vi "EvaluateNode.vi"(8 "error in (no error)":errorcluster, 10 "ToEvaluate in":refnum<data-value>, 11 "Graph in":refnum<class "Graph.lvclass">) -> (0 "error out":errorcluster, 2 "ToEvaluate out":refnum<data-value>, 3 "Graph out":refnum<class "Graph.lvclass">)   [LabVIEW 2014, in "Graph.lvlib" / "Graph.lvclass"]
doc: "Calls the Evaluation method of a node, then applies the value to the node, then sets the ToSortBy so it can be placed in OPEN."
uses:
  <userlib>/AdvancedDataStructures/ClassBased/Graph/Graph.lvclass
  <userlib>/AdvancedDataStructures/ClassBased/GraphNode/GraphNode.lvclass
  <userlib>/AdvancedDataStructures/ClassBased/Common/BasicSortedList/BasicSortedNode/BasicSortedNode.lvclass
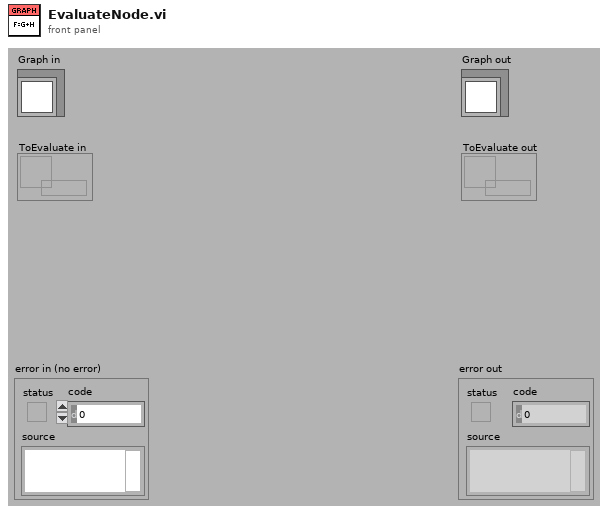
[diagram p1: front panel]
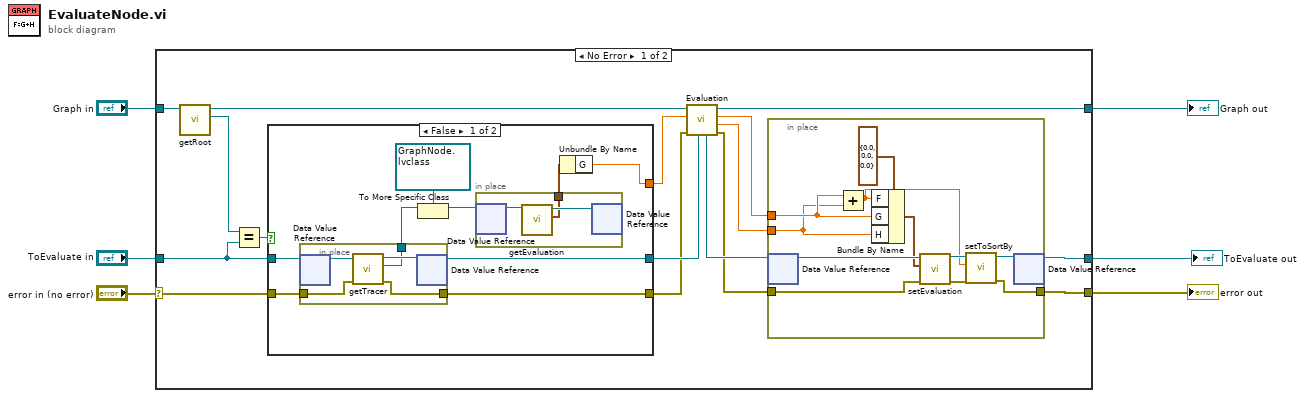
[diagram p0: block diagram]
diagram:
  n1 = case shown="No Error" "error in (no error)" {
    selector: "error in (no error)" -> [w18 w55]
    tunnel: [w8 w55] -> w5
    tunnel: [w7 w54] -> w3
    tunnel: "Graph in" -> [w22 w54]
    tunnel: "ToEvaluate in" -> [w19 w53]
    tunnel: [w9 w53] -> w1
    frame No Error {
      n2 = call <userlib>:"getRoot.vi"("Graph in"=w22) -> ("Root"=w21:refnum<data-value>, "Graph out"=w17:refnum<class "Graph.lvclass">)  [unwired: 8 in, 1 out]
      n3 = Equal?(x=w21, y=w19) -> (x = y?=w20:bool)
      n4 = case shown="False" w20 {
        tunnel: w19 -> [w42 w52]
        tunnel: [w39 w52] -> w15
        tunnel: w18 -> [w41 w51]
        tunnel: [w40 w51] -> w14
        tunnel: [w35 _] -> w16
        frame False {
          n5 = in-place {
            in-place-border: [w48] -> w38
            in-place-border: w41 -> [w47]
            in-place-border: [w46] -> w40
            n6 = in-place-dvr #1(w42) -> (w50:refnum<class "GraphNode.lvclass">)  [unwired: 1 out]
            n7 = call <userlib>:"getTracer.vi"("error in (no error)"=w47, "GraphNode in"=w50) -> ("error out"=w46:errorcluster, "tracer"=w48:refnum<data-value>, "GraphNode out"=w49:refnum<class "GraphNode.lvclass">)  [unwired: 7 in]
            n8 = in-place-dvr #1(w49) -> (w39:refnum<data-value>)  [unwired: 1 out]
          }
          n9 = To More Specific Class(target class=refnum<data-value> refnum ("ToEvaluate in"), reference=w38) -> (specific class reference=w36:refnum<data-value>)  [unwired: 1 in, 1 out]
          n10 = in-place {
            in-place-border: [w43] -> w34
            n11 = in-place-dvr #2(w36) -> (w45:refnum<class "GraphNode.lvclass">)  [unwired: 1 out]
            n12 = call <userlib>:"getEvaluation.vi"("GraphNode in"=w45) -> ("Evaluation"=w43:cluster{"F":dbl, "G":dbl, "H":dbl}, "GraphNode out"=w44:refnum<class "GraphNode.lvclass">)  [unwired: 8 in, 1 out]
            n13 = in-place-dvr #2(w44) -> ()  [unwired: 2 out]
          }
          n14 = Unbundle By Name(w34) -> ("G"=w35:dbl)
        }
        frame True {
        }
      }
      n15 = call-dynamic "Evaluation.vi"("ToEvaluate in"=w15, "error in (no error)"=w14, "Parents G"=w16, "Graph in"=w17) -> ("error out"=w10:errorcluster, "H"=w11:dbl, "G"=w12:dbl, "Graph out"=w7:refnum<class "Graph.lvclass">, "ToEvaluate out"=w13:refnum<data-value>)  [unwired: 3 in]
      n16 = in-place {
        in-place-border: w12 -> [w32]
        in-place-border: w11 -> [w31]
        in-place-border: w10 -> [w25]
        in-place-border: [w23] -> w8
        n17 = in-place-dvr #3(w13) -> (w30:refnum<class "GraphNode.lvclass">)  [unwired: 1 out]
        n18 = Add(x=w32, y=w31) -> (x+y=w26:dbl)
        n19 = Bundle By Name(cluster=cluster{"F":dbl, "G":dbl, "H":dbl} {"F"=0.0, "G"=0.0, "H"=0.0} ("evaluation"), "F"=w26, "G"=w32, "H"=w31) -> (w29:cluster{"F":dbl, "G":dbl, "H":dbl})
        n20 = call <userlib>:"setEvaluation.vi"("error in (no error)"=w25, "Evaluation"=w29, "GraphNode in"=w30) -> ("error out"=w24:errorcluster, "GraphNode out"=w28:refnum<class "GraphNode.lvclass">)  [unwired: 7 in]
        n21 = call <userlib>:"setToSortBy.vi"("error in (no error)"=w24, "ToSortBy"=w26, "BasicSortedNode in"=w28) -> ("error out"=w23:errorcluster, "BasicSortedNode out"=w27:refnum<class "GraphNode.lvclass">)  [unwired: 7 in]
        n22 = in-place-dvr #3(w27) -> (w9:refnum<data-value>)  [unwired: 1 out]
      }
    }
    frame Error {
    }
  }
  "error out" <- w5
  "Graph out" <- w3
  "ToEvaluate out" <- w1
